vi "UpdateProgramStatus.vi"(0 "Program Interface in":refnum<class "Program Interface.lvclass">, 1 "Program Status in":T1, 5 "error in (no error)":errorcluster) -> (14 "Program Interface out":refnum<class "Program Interface.lvclass">, 15 "Program Status out":T1, 19 "error out":errorcluster)   [LabVIEW 2016, in "Program Interface.lvclass"]
uses:
  Program Interface.lvclass
  Robot/Universal Robot/ProgramStatus.ctl
  Robot/Universal Robot/ProgramState.ctl
  Program Interface.lvclass/Program Interface.ctl
  Robot/Universal Robot/Universal Robot.lvclass
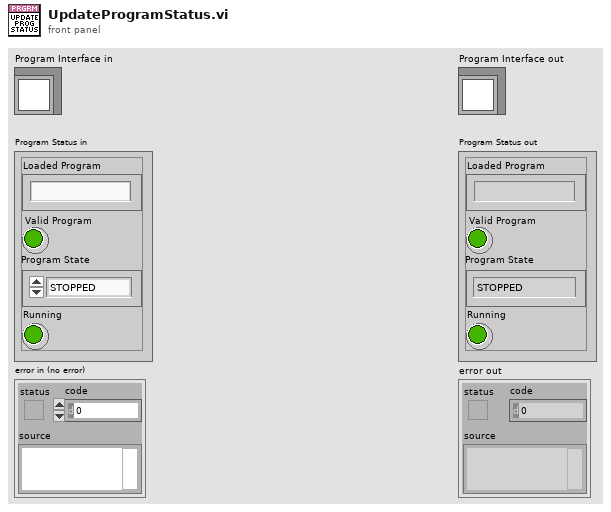
[diagram p1: front panel]
types:
  T1 = typedef "Universal Robot.lvclass/ProgramStatus.ctl" = cluster{"Loaded Program":string, "Valid Program":bool, "Program State":T2, "Running":bool}
  T2 = typedef "Universal Robot.lvclass/ProgramState.ctl" = enum16{"STOPPED", "PLAYING", "PAUSE"}
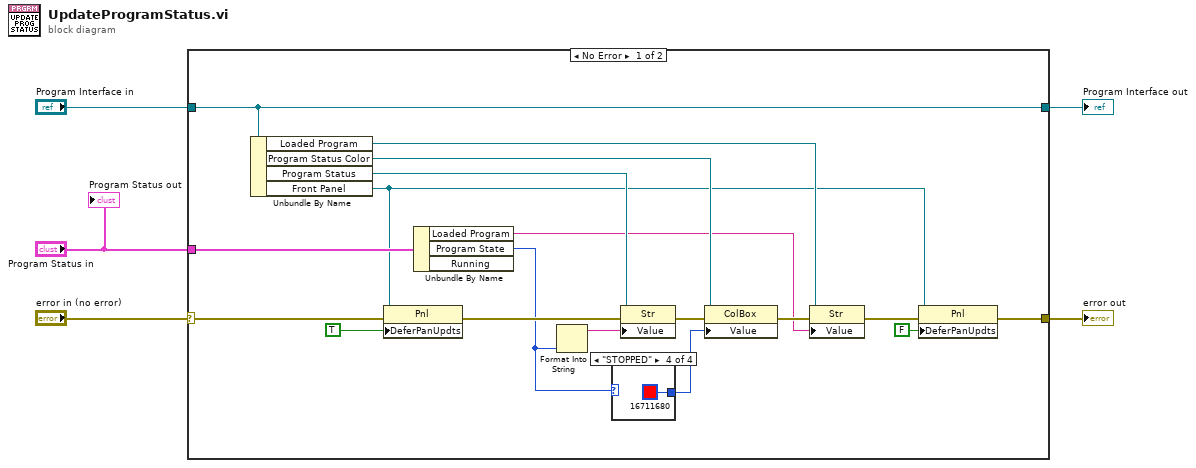
[diagram p0: block diagram]
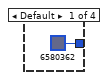
[diagram p2: hidden frame]
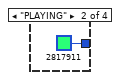
[diagram p3: hidden frame]
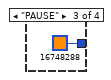
[diagram p4: hidden frame]
diagram:
  n1 = case shown="No Error" "error in (no error)" {
    selector: "error in (no error)" -> [w16 w29]
    tunnel: [w11 w29] -> w4
    tunnel: [w23 w28] -> w2
    tunnel: "Program Interface in" -> [w23 w28]
    tunnel: "Program Status in" -> [w22 _]
    frame No Error {
      n2 = Unbundle By Name(w23) -> ("Loaded Program"=w17:refnum<vi>, "Program Status Color"=w19:refnum<vi>, "Program Status"=w21:refnum<vi>, "Front Panel"=w12:refnum<vi>)
      n3 = property class="Pnl"(reference=w12, error in=w16, "DeferPanUpdts"=TRUE ("Defer Panel Updates")) -> (error out=w15:errorcluster)  [unwired: 1 out]
      n4 = Unbundle By Name(w22) -> ("Loaded Program"=w7:string, "Program State"=w10:T2)  [unwired: 1 out]
      n5 = Format Into String(w10) -> (resulting string=w8:string)  [unwired: 3 in, 1 out]
      n6 = case shown="\"STOPPED\"" w10 {
        tunnel: [u32 6580362 u32 2817911 u32 16748288 u32 16711680] -> w9
        frame Default {
        }
        frame "PLAYING" {
        }
        frame "PAUSE" {
        }
        frame "STOPPED" {
        }
      }
      n7 = property class="Str"(reference=w21, error in=w15, "Value"=w8) -> (error out=w20:errorcluster)  [unwired: 1 out]
      n8 = property class="ColBox"(reference=w19, error in=w20, "Value"=w9) -> (error out=w18:errorcluster)  [unwired: 1 out]
      n9 = property class="Str"(reference=w17, error in=w18, "Value"=w7) -> (error out=w6:errorcluster)  [unwired: 1 out]
      n10 = property class="Pnl"(reference=w12, error in=w6, "DeferPanUpdts"=FALSE ("Defer Panel Updates")) -> (error out=w11:errorcluster)  [unwired: 1 out]
    }
    frame Error {
    }
  }
  "error out" <- w4
  "Program Interface out" <- w2
  "Program Status out" <- "Program Status in"
